vi "check_for_execution_stop_test.vi"() -> ()   [LabVIEW 2017, in "labview-standard-library.lvlib" / "automode-scripting.lvlib"]
uses:
  automode-scripting.lvlib
  type-defs/execution_stop_type.ctl
panel:
  out "All passing?":bool
  out "Stop type":bool[](array[boolean])
  out "millisecond wait":bool[](array[boolean])
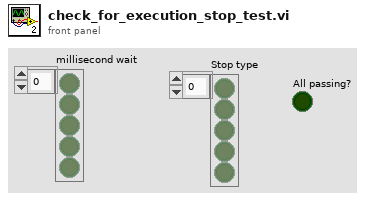
[diagram p1: front panel]
types:
  T1 = typedef "execution_stop_type.ctl" = u16
  T2 = typedef "labview-standard-library.lvlib/automode-scripting.lvlib/execution_stop_type.ctl" = enum16{"G4 timed pause", "G4 all execution pause", "G4 single execution pause", "M0 Breakpoint", "Invalid"}
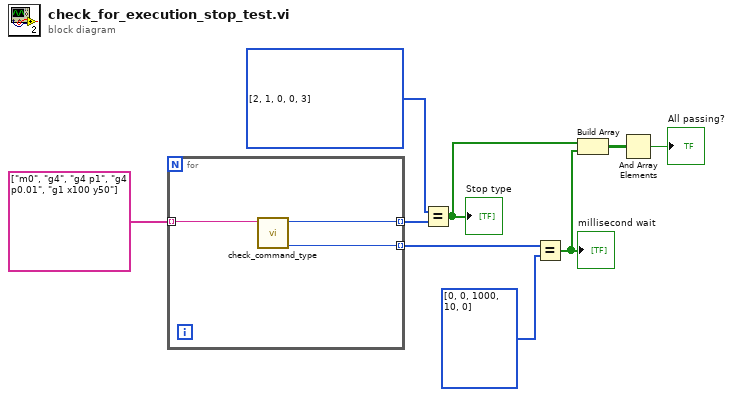
[diagram p0: block diagram]
diagram:
  w8 = T1[] [2, 1, 0, 0, 3] items=["G4 timed pause", "G4 execution pause", "M0 Breakpoint", "None"]
  n1 = for {
    tunnel: string[] ["m0", "g4", "g4 p1", "g4 p0.01", "g1 x100 y50"] -> [w12] mode=indexing
    tunnel: [w11] -> w7 mode=indexing
    tunnel: [w10] -> w6 mode=indexing
    n2 = call "check_command_type.vi"("Current command"=w12) -> ("Wait for: __ milliseconds"=w10:u32, "stop type"=w11:T2)  [unwired: 9 in]
  }
  n3 = Equal?(x=w8, y=w7) -> (x = y?=w4:bool[])
  "Stop type" <- w4
  n4 = Equal?(x=w6, y=u32[] [0, 0, 1000, 10, 0]) -> (x = y?=w3:bool[])
  "millisecond wait" <- w3
  n5 = Build Array(w4, w3) -> (w2:bool[][])
  n6 = And Array Elements(Boolean array=w2) -> (logical AND=→"All passing?":bool)
